vi "Calibrate In Ear.vi"(9 "Auto cal (F)?":bool, 11 "State":T1) -> (0 "error out":errorcluster)   [LabVIEW 2020]
uses:
  Utility VIs/Type Defs/Speaker ring.ctl
  Utility VIs/Buttons/KCheckmarkBoolean 2.ctl
  Cochlear Function Test Suite/LV Source/CFTS Main Panel SubVIs/CFTS-Experiment State.ctl
  Type Defs/ACal-In Ear Parameters.ctl
  Type Defs/Cal Stimulus.ctl
  Type Defs/ACal-Multiband Parameters.ctl
  Utility VIs/Conversion VIs/Create Waveform Cluster (2D).vi
  Utility VIs/Math VIs/FFT x(t) to dB,Degrees (2D).vi
  Instance           1 24Saved   Calibrate In Ear .vi
  Utility VIs/File IO VIs/Configuration File Wrapper VIs/Config-Read Key (Boolean).vi
panel:
  in  "Weighted":bool
  out "Auto Message":string="Auto calibrating!"
  in  "Speaker":T2
  in  "mic gain":dbl caption="Probe Mic Gain (dB)"
  in  "Stimulus":T3={"Min Freq (Hz)"=1000.0, "Max Freq (Hz)"=50000.0, "Freq Step (Hz)"=50.0, "Waveform"=0, "Attenuation (dB)"=30.0, "Sample Rate (Hz)"=100000.0} {"Waveform" items=["Chirp"]}
  out "Stimulus graph":cluster{i32, dbl, dbl[]}(graph)={0, 0.01, []}
  in  "Averages":i32=128
  in  "Return":bool
  in  "START":bool
  in  "STOP":bool
  out "Path":path
  in  "Data tab":enum32{"Raw", "Calibration"}(tab)
  out "Mic signals":cluster{"offset":dbl, "dx":dbl, "Y":dbl[][]}(graph)
  out "Mic mag":cluster{"offset":dbl, "dx":dbl, "Y":dbl[][]}(graph)
  out "Acquired":i32=256
  in  "Clear":bool
  in  "Load":bool
  in  "Show all":bool
  in  "Last N":bool
  out "ASTF":cluster{"Frequency":dbl[], "Frequency":dbl[]}[](graph)
  in  "Plot Max SPL":T4=TRUE
  in  "result":cluster{"Path":path, "error ":errorcluster}
  out "ASTF phase":cluster{"Frequency":dbl[], "Frequency":dbl[]}[](graph)
  out "Mic phase graph":cluster{"offset":dbl, "dx":dbl, "Y":dbl[][]}(graph)
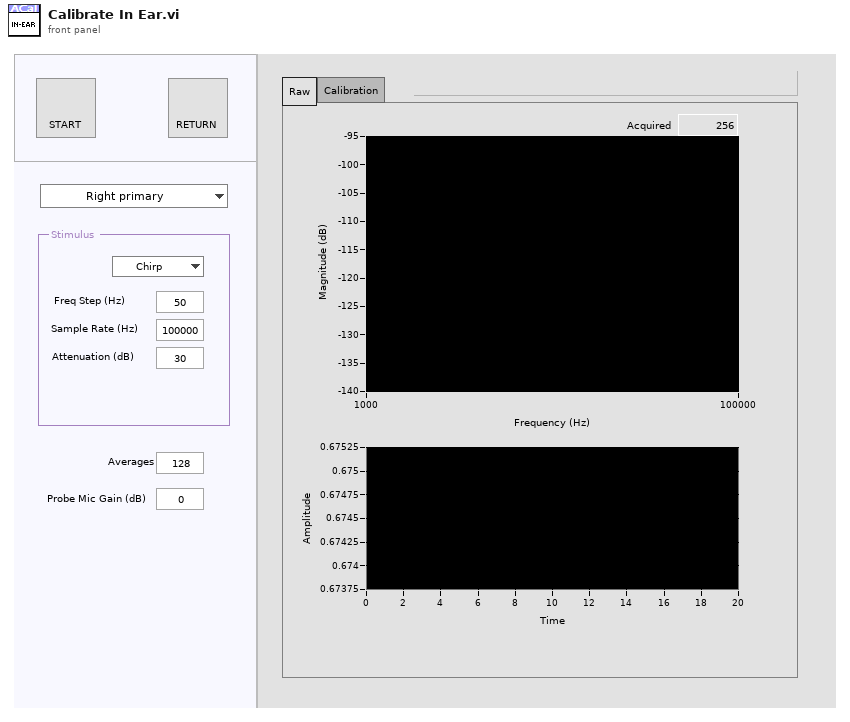
[diagram p1: front panel]
types:
  T1 = typedef "CFTS-Experiment State.ctl" = cluster{"Experimenter":string, "Number":u32, "Right":string, "Left":string, "Data Folder":path, "State File":path, "Version Info":string, "End Exposure Time":dbl, "Exposure Duration":string, "Run #":cluster{"CAP":i16, "ABR":i16, "DP":i16, "VsEP":i16, "MeasSeq":i16, "SubSeq":i16, "SFOAE":i16}}
  T2 = typedef "Speaker ring.ctl" = enum16{"Right primary", "Right secondary", "Left primary", "Left secondary"}
  T3 = cluster{"Min Freq (Hz)":dbl, "Max Freq (Hz)":dbl, "Freq Step (Hz)":dbl, "Waveform":u16, "Attenuation (dB)":dbl, "Sample Rate (Hz)":dbl}
  T4 = typedef "KCheckmarkBoolean 2.ctl" = bool
  T5 = typedef "ACal-In Ear Parameters.ctl" = cluster{"Speaker":T2, "Stimulus":T6, "Averages":i32, "Left gain":dbl, "Right gain":dbl, "plot max":bool, "smooth override":bool, "Weighted":T7, "Max Vmic":dbl}
  T6 = typedef "Cal Stimulus.ctl" = cluster{"Min Freq (Hz)":dbl, "Max Freq (Hz)":dbl, "Freq Step (Hz)":dbl, "Waveform":enum16{"Chirp", "Weighted"}, "Attenuation (dB)":dbl, "Sample Rate (Hz)":dbl}
  T7 = typedef "ACal-Multiband Parameters.ctl" = cluster{"Folder":path, "Fmin":dbl, "Fmax":dbl, "Max range":dbl, "WF":u16}
  T8 = typedef "Cal-Smoothing Parameters.ctl" = cluster{"Method":enum16{"None", "Moving average", "Loess"}, "MA":cluster{"Iterations":i32, "Length":i32}, "Loess":cluster{"Length":i32, "Type":enum16{"Linear", "Quadratic"}, "Robust":bool}}
  T9 = cluster{"new file path":path, "error out":errorcluster}
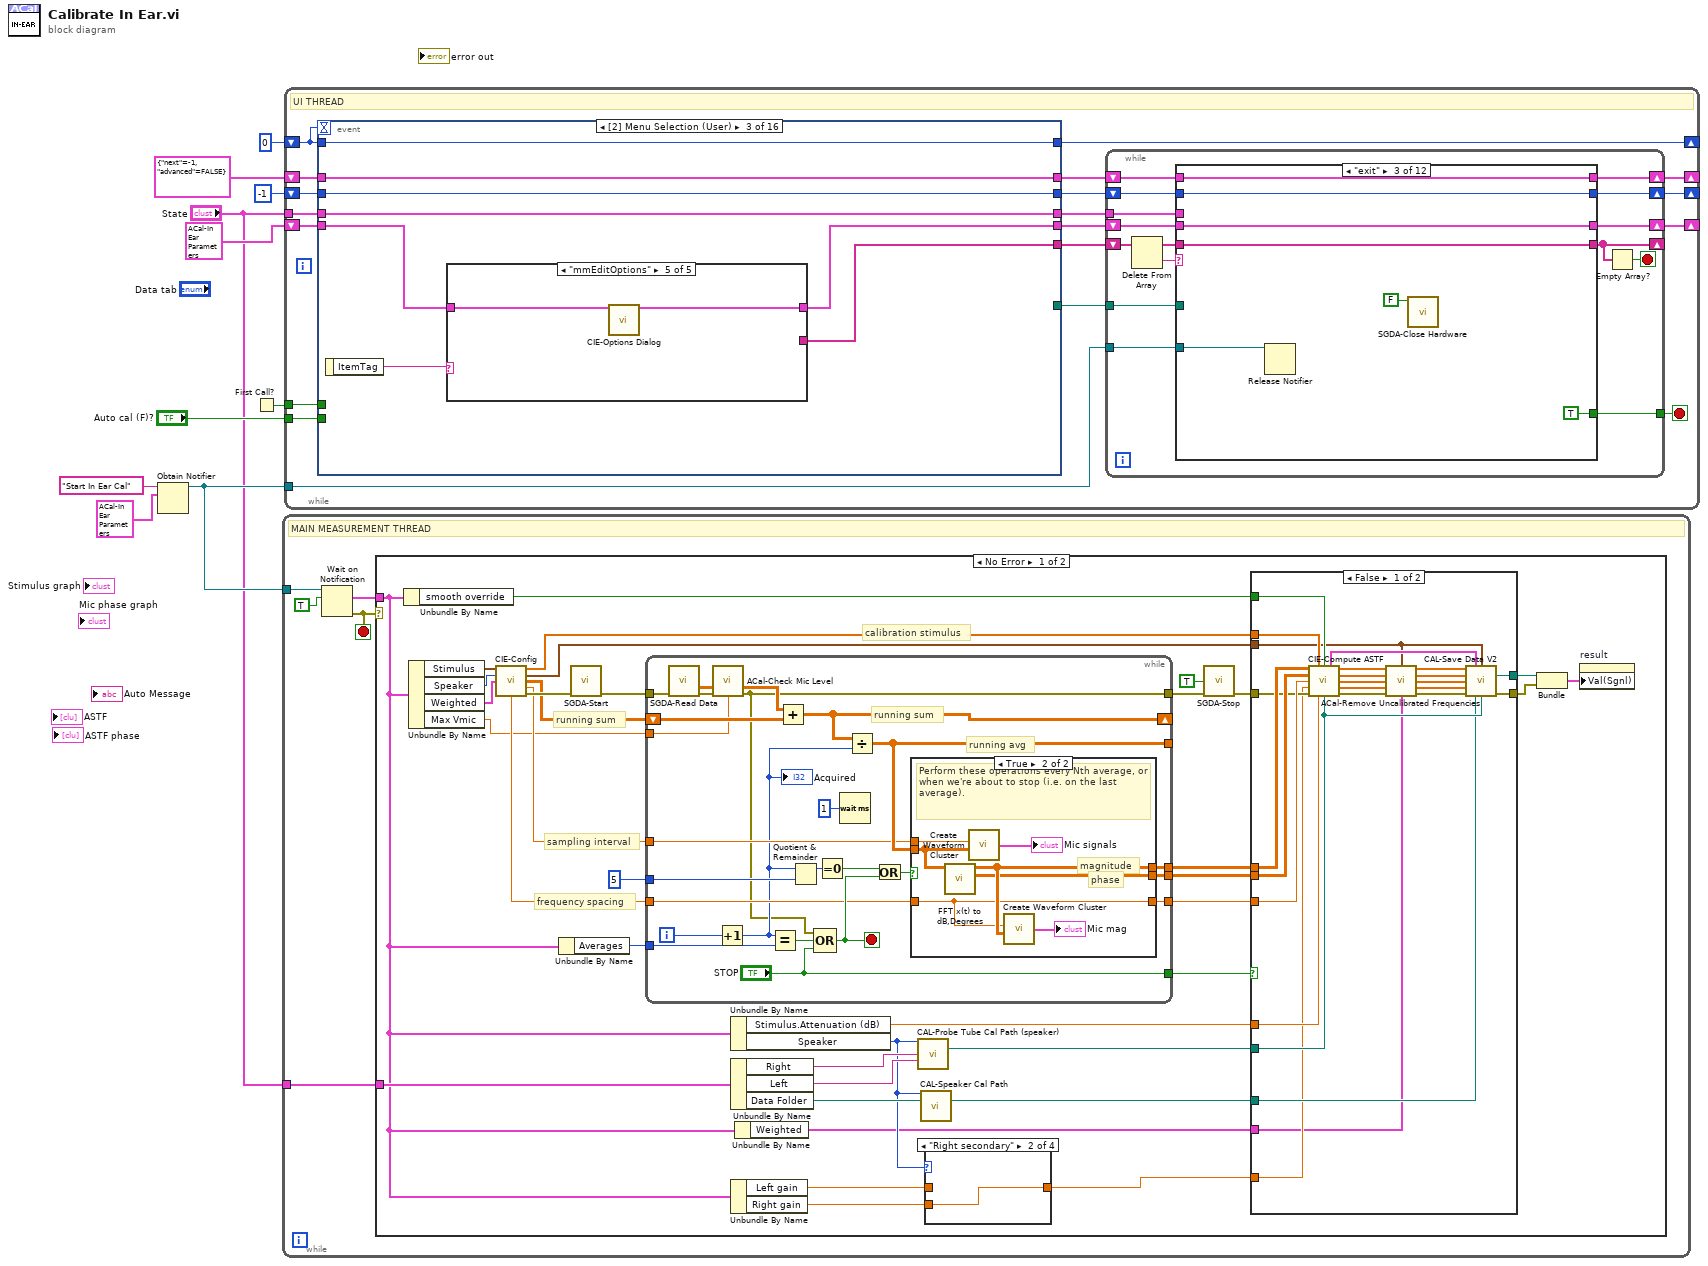
[diagram p0: block diagram]
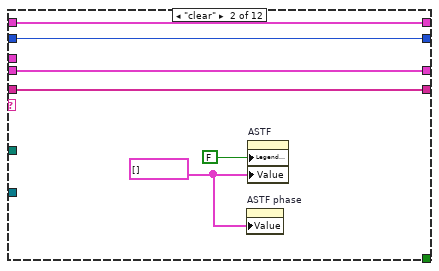
[diagram p9: hidden frame]
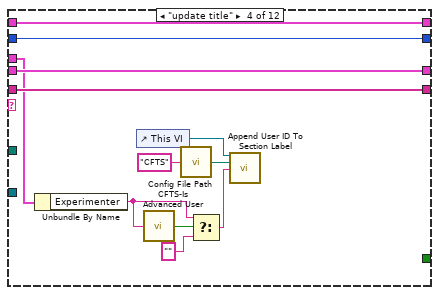
[diagram p10: hidden frame]
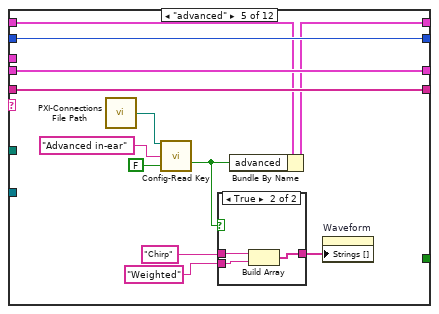
[diagram p11: hidden frame]
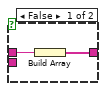
[diagram p12: hidden frame]
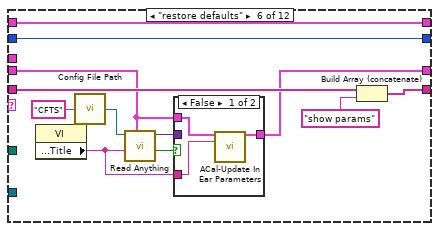
[diagram p13: hidden frame]
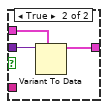
[diagram p14: hidden frame]
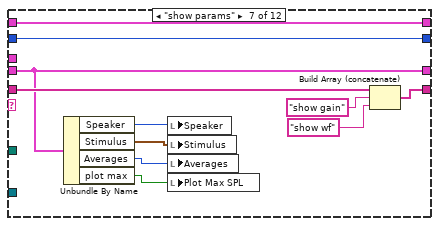
[diagram p15: hidden frame]
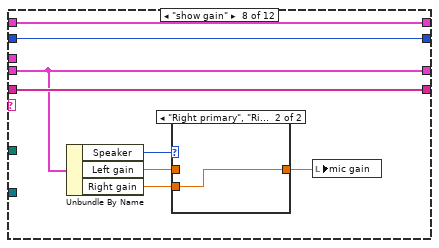
[diagram p16: hidden frame]
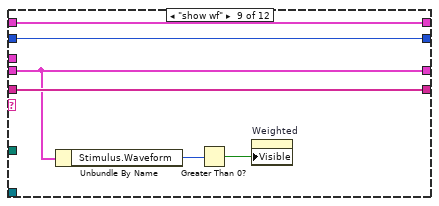
[diagram p18: hidden frame]
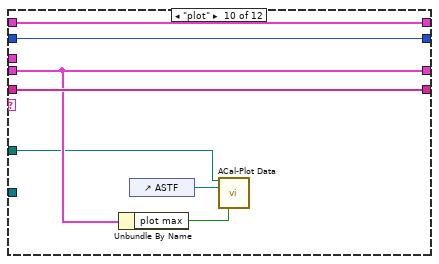
[diagram p19: hidden frame]
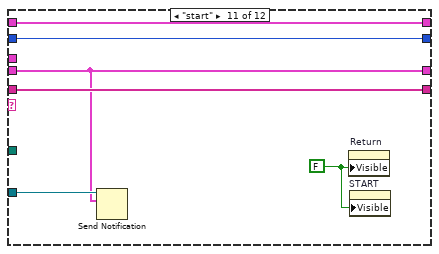
[diagram p20: hidden frame]
diagram:
  n1 = Obtain Notifier(name (unnamed)="Start In Ear Cal", notification data type=T5 {"Speaker"=enum."Right primary", "Stimulus"={"Min Freq (Hz)"=50.0, "Max Freq (Hz)"=50000.0, "Freq Step (Hz)"=50.0, "Waveform"=enum."Chirp", "Attenuation (dB)"=20.0, "Sample Rate (Hz)"=100000.0}, "Averages"=512, "Left gain"=40.0, "Right gain"=40.0, "plot max"=TRUE, "smooth override"=FALSE, "Weighted"={"Folder"=path "", "Fmin"=0.0, "Fmax"=0.0, "Max range"=0.0, "WF"=0}, "Max Vmic"=0.0} ("Params")) -> (notifier out=w10:refnum<notifier>)  [unwired: 2 in, 2 out]
  n2 = First Call?() -> (First Call?: T/F=w1:bool)
  n3 = while {
    tunnel: w10 -> [w15]
    tunnel: "State" -> [w13]
    stop <- w14 stop-if-true
    # "MAIN MEASUREMENT THREAD"
    n4 = Wait on Notification(notifier=w15, ignore previous (F)=TRUE) -> (notification=w12:T5, error out=w14:errorcluster)  [unwired: 2 in, 2 out]
    n5 = case shown="No Error" w14 {
      tunnel: w13 -> [w34 _]
      tunnel: w12 -> [w19 _]
      frame No Error {
        # "calibration stimulus"
        # "frequency spacing"
        # "sampling interval"
        # "running sum"
        n6 = Unbundle By Name(w19) -> ("smooth override"=w30:bool)
        n7 = Unbundle By Name(w19) -> ("Stimulus"=w33:T6, "Speaker"=w32:T2, "Weighted"=w20:T7, "Max Vmic"=w17:dbl)
        n8 = call "CIE-Config.vi"("Cal Stimulus"=w33, "Speaker"=w32, "Weighted"=w20) -> ("Stimulus"=w45:dbl[], "Cal Spec Out"=w36:T6, "Mic Avg"=w51:dbl[][], "dt (ms)"=w49:dbl, "df (Hz)"=w50:dbl, "error out"=w52:errorcluster)  [unwired: 6 in, 1 out]
        n9 = Unbundle By Name(w19) -> ("Averages"=w31:i32)
        n10 = call "SGDA-Start.vi"("error in (no error)"=w52) -> ("error out"=w44:errorcluster)  [unwired: 6 in]
        n11 = while {
          tunnel: w44 -> [w107]
          tunnel: [w83] -> w43
          tunnel: w31 -> [w104]
          shift-right: [w102] -> _
          shift-left: w51 -> [w103]
          tunnel: [w101] -> _
          tunnel: 5 -> [w100]
          tunnel: w50 -> [w95]
          tunnel: [w94] -> w48
          tunnel: [w93] -> w47
          tunnel: w49 -> [w92]
          tunnel: [w91] -> w46
          tunnel: ["STOP"] -> w28
          tunnel: w17 -> [w84]
          i -> [w106]
          stop <- w96 stop-if-true
          # "running avg"
          # "running sum"
          n12 = call "SGDA-Read Data.vi"("error in (no error)"=w107) -> ("AI Waveforms"=w86:dbl[][], "error out"=w87:errorcluster)  [unwired: 13 in]
          n13 = call "ACal-Check Mic Level.vi"("AI Waveforms in"=w86, "error in (no error)"=w87, "Max Vmic"=w84) -> ("AI Waveforms out"=w85:dbl[][], "error out"=w83:errorcluster)  [unwired: 11 in]
          n14 = Increment(x=w106) -> (x+1=w90:i32)
          "Acquired" <- w90
          n15 = Equal?(x=w90, y=w104) -> (x = y?=w105:bool)
          n16 = Add(x=w85, y=w103) -> (x+y=w102:dbl[][])
          n17 = Quotient & Remainder(x=w90, y=w100) -> (x-y*floor(x/y)=w99:i32)  [unwired: 1 out]
          n18 = Compound Arithmetic op=OR(w83, w105, "STOP") -> (w96:bool)
          n19 = Equal To 0?(x=w99) -> (x = 0?=w97:bool)
          n20 = Wait (ms)(milliseconds to wait=u32 1) -> ()  [unwired: 1 out]
          n21 = Divide(x=w102, y=w90) -> (x/y=w101:dbl[][])
          n22 = Or(x=w97, y=w96) -> (x .or. y?=w98:bool)
          n23 = case shown="True" w98 {
            tunnel: w101 -> [_ w111]
            tunnel: w95 -> [_ w108]
            tunnel: [_ w113] -> w94
            tunnel: [_ w112] -> w93
            tunnel: w92 -> [_ w110]
            tunnel: [_ w108] -> w91
            frame False {
            }
            frame True {
              # "phase"
              # "magnitude"
              # "Perform these operations every Nth average, or when we're about to stop (i.e. on the last average)."
              n24 = call-poly "FFT x(t) to dB,Degrees.vi"("X(t)"=w111) -> ("+Freq Phase of FFT (degrees)"=w112:dbl[][], "+Freq. Mag of FFT (dB rms)"=w113:dbl[][])  [unwired: 9 in]
              n25 = call-poly "Create Waveform Cluster.vi"("dx"=w110, "Array"=w111) -> ("waveform cluster"=→"Mic signals":cluster{"offset":dbl, "dx":dbl, "Y":dbl[][]})  [unwired: 3 in]
              n26 = call-poly "Create Waveform Cluster.vi"("dx"=w108, "Array"=w113) -> ("waveform cluster"=→"Mic mag":cluster{"offset":dbl, "dx":dbl, "Y":dbl[][]})  [unwired: 3 in]
            }
          }
        }
        n27 = Unbundle By Name(w19) -> ("Stimulus.Attenuation (dB)"=w29:dbl, "Speaker"=w27:T2)
        n28 = Unbundle By Name(w34) -> ("Right"=w41:string, "Left"=w40:string, "Data Folder"=w39:path)
        n29 = Unbundle By Name(w19) -> ("Left gain"=w26:dbl, "Right gain"=w24:dbl)
        n30 = Unbundle By Name(w19) -> ("Weighted"=w18:T7)
        n31 = call "CAL-Probe Tube Cal Path (speaker).vi"("Speaker"=w27, "Right"=w41, "Left"=w40) -> ("Probe Tube Cal Path"=w38:path)  [unwired: 11 in, 1 out]
        n32 = call "CAL-Speaker Cal Path.vi"("Speaker"=w27, "Data Folder"=w39) -> ("Cal Path"=w35:path)  [unwired: 12 in, 1 out]
        n33 = case shown="\"Right secondary\"" w27 {
          tunnel: w26 -> [_ _ w55 w56]
          tunnel: [w53 w54 w55 w56] -> w25
          tunnel: w24 -> [w53 w54 _ _]
          frame "Right primary", Default {
          }
          frame "Right secondary" {
          }
          frame "Left secondary" {
          }
          frame "Left primary" {
          }
        }
        n34 = call "SGDA-Stop.vi"("Clear ActiveX (F)"=TRUE, "error in (no error)"=w43) -> ("error out"=w37:errorcluster)  [unwired: 13 in]
        n35 = case shown="False" w28 {
          tunnel: w48 -> [w81 _]
          tunnel: w47 -> [w80 _]
          tunnel: w46 -> [w79 _]
          tunnel: w45 -> [w78 _]
          tunnel: w38 -> [w77 _]
          tunnel: w37 -> [w76 w82]
          tunnel: w36 -> [w58 _]
          tunnel: w35 -> [w74 _]
          tunnel: w30 -> [w73 _]
          tunnel: w29 -> [w72 _]
          tunnel: [w71 w82] -> w22
          tunnel: [w70 _] -> w23
          tunnel: w25 -> [w69 _]
          tunnel: w18 -> [w57 _]
          frame False {
            n36 = call "CIE-Compute ASTF.vi"("Mag"=w81, "Stimulus"=w78, "Force no smoothing?"=w73, "Phase"=w80, "df (Hz)"=w79, "Probe Mic Gain (dB)"=w69, "error in (no error)"=w76, "Attenuation (dB)"=w72, "Probe Tube Path"=w77) -> ("Smooth Params"=w75:T8, "ASTF Mag"=w60:dbl[], "ASTF Phase"=w61:dbl[], "Frequency"=w64:dbl[], "Unsmoothed Mag"=w65:dbl[], "error out"=w68:errorcluster)  [unwired: 1 in]
            n37 = call "ACal-Remove Uncalibrated Frequencies.vi"("ASTF Mag in"=w60, "Cal Spec Out"=w58, "ASTF Phase in"=w61, "Frequency in"=w64, "Unsmoothed Mag in"=w65, "error in (no error)"=w68, "Weighted"=w57) -> ("ASTF Mag out"=w59:dbl[], "ASTF Phase out"=w62:dbl[], "Frequency out"=w63:dbl[], "Unsmoothed Mag out"=w66:dbl[], "error out"=w67:errorcluster)  [unwired: 4 in]
            n38 = call "CAL-Save Data V2.vi"("Mag"=w59, "Smooth Params"=w75, "Cal Stimulus"=w58, "Phase"=w62, "Frequency"=w63, "Unsmoothed Mag"=w66, "error in (no error)"=w67, "path"=w74, "Probe Tube File"=w77) -> ("new file path"=w70:path, "error out"=w71:errorcluster)  [unwired: 5 in]
          }
          frame True {
          }
        }
        n39 = Bundle("new file path"=w23, "error out"=w22) -> (w21:T9)  [unwired: 1 in]
        n40 = property on="result" class="Clust (strict)"("Val(Sgnl)"=w21) -> ()  [unwired: 2 in, 2 out]
      }
      frame Error {
      }
    }
  }
  n41 = while {
    tunnel: w10 -> [w121]
    shift-right: [w130] -> _
    shift-left: 0 -> [w131]
    tunnel: "Auto cal (F)?" -> [w133]
    shift-right: [w124] -> _
    shift-left: -1 -> [w132]
    tunnel: "State" -> [w129]
    shift-right: [w125] -> _
    shift-left: T5 {"Speaker"=enum."Right primary", "Stimulus"={"Min Freq (Hz)"=50.0, "Max Freq (Hz)"=50000.0, "Freq Step (Hz)"=50.0, "Waveform"=enum."Chirp", "Attenuation (dB)"=20.0, "Sample Rate (Hz)"=100000.0}, "Averages"=512, "Left gain"=40.0, "Right gain"=40.0, "plot max"=TRUE, "smooth override"=FALSE, "Weighted"={"Folder"=path "C:/Data", "Fmin"=3000.0, "Fmax"=45000.0, "Max range"=25.0, "WF"=0}, "Max Vmic"=0.0} ("Params") -> [w128]
    shift-right: [w116] -> _
    shift-left: cluster{"next":i32, "advanced":bool} {"next"=-1, "advanced"=FALSE} -> [w118]
    tunnel: w1 -> [w115]
    stop <- w122 stop-if-true
    # "UI THREAD"
    n42 = event shown="[2] Menu Selection (User)" {
      selector: _ -> [_ _ _ _ _ _ _ _ _ _ _ _ _ _ _ _]
      dyn-events: _ -> [_ _ _ _ _ _ _ _ _ _ _ _ _ _ _ _]
      timeout: w131 -> [_ _ _ _ _ _ _ _ _ _ _ _ _ _ _ _]
      tunnel: w133 -> [w288 _ _ _ _ _ _ _ _ _ _ w411 _ _ _ _]
      tunnel: w132 -> [w289 w306 w315 w335 w342 w350 w353 w366 w368 w381 w394 w419 w435 w442 w457 w467]
      tunnel: [w289 w306 w315 w335 w342 w350 w353 w366 w368 w381 w394 w419 w435 w442 w457 w467] -> w127
      tunnel: w131 -> [_ w305 w314 w334 w341 w349 w358 w365 w373 w380 w393 w418 w434 w441 w455 w465]
      tunnel: [-1 w305 w314 w334 w341 w349 w358 w365 w373 w380 w393 w418 w434 w441 w455 w465] -> w130
      tunnel: w129 -> [w284 w302 w309 w331 w340 w344 w356 w364 w371 w376 w391 w416 w431 w439 w454 w464]
      tunnel: w128 -> [w286 w304 w312 w333 w339 w348 w357 w362 w372 w378 w392 w417 w433 w440 w453 w463]
      tunnel: [w286 w304 w311 w333 w339 w346 w355 w360 w370 w377 w390 w417 w433 w440 w453 w463] -> w126
      tunnel: [w283 string[] ["exit"] w310 string[] ["exit"] string[] ["start"] string[] ["show gain"] string[] ["show wf"] _ _ _ _ w409 string[] ["clear"] w437 _ _] -> w123
      tunnel: [w284 w302 w309 w331 w340 w344 w356 w364 w371 w376 w391 w416 w431 w439 w454 w464] -> w120
      tunnel: [_ _ _ _ _ _ _ _ _ _ _ w414 _ w438 _ _] -> w119
      tunnel: w118 -> [w281 w301 w308 w330 w338 w343 w352 w363 w367 w374 w388 w413 w430 w436 w451 w460]
      tunnel: [w281 w301 w308 w330 w338 w343 w352 w363 w367 w374 w388 w413 w430 w436 w451 w460] -> w117
      tunnel: w115 -> [w279 _ _ _ _ _ _ _ _ _ _ _ _ _ _ _]
      event Timeout {
        w295 = TRUE ("Visible")
        n43 = event-data() -> ()  [unwired: 1 in, 1 out]
        n44 = call "SGDA-Initialize Hardware.vi"("Start PXI Server"=FALSE) -> ()  [unwired: 13 in, 2 out]
        n45 = case shown="False" w288 {
          tunnel: [w297 string[] ["next", "clear"]] -> w285
          tunnel: w279 -> [w299 _]
          frame False {
            n46 = Select(t=string[] ["clear"], s=w299, f=string[] []) -> (s? t:f=w297:string[])
          }
          frame True {
          }
        }
        n47 = property on="Auto Message" class="Str"("Visible"=w288, "Blinking"=w288) -> ()  [unwired: 2 in, 2 out]
        n48 = Unbundle By Name(w284) -> ("Experimenter"=w294:string)
        n49 = property on="Weighted" class="Bool"("Visible"=FALSE) -> ()  [unwired: 2 in, 2 out]
        n50 = Concatenate Strings(w294, ": Last 5" ("string")) -> (w292:string)
        n51 = property on="START" class="Bool"("Visible"=w295) -> ()  [unwired: 2 in, 2 out]
        n52 = property on="Return" class="Bool"("Visible"=w295) -> ()  [unwired: 2 in, 2 out]
        n53 = Initialize Array(w292, 4 ("dimension size")) -> (w290:string[])
        n54 = property on="Last N" class="Bool"("Strings [4]"=w290) -> ()  [unwired: 2 in, 2 out]
        n55 = Build Array (concatenate)(w285, string[] ["restore defaults", "advanced", "update title"]) -> (w283:string[])
      }
      event Panel Close? {
        n56 = event-data() -> ()  [unwired: 1 in, 1 out]
        n57 = event-data("Discard?"=TRUE) -> ()  [unwired: 1 in, 1 out]
      }
      event Menu Selection (User) {
        n58 = event-data() -> ("ItemTag"=w313:string)  [unwired: 1 in]
        n59 = case shown="\"mmEditOptions\"" w313 {
          tunnel: w312 -> [w316 w318 w321 w327 w329]
          tunnel: [w316 w318 w321 w327 w328] -> w311
          tunnel: [_ string[] ["restore defaults"] _ string[] ["exit"] _] -> w310
          frame "", Default {
          }
          frame "mmFileRestore" {
          }
          frame "mmFileSave" {
            n60 = property class="VI"() -> ("Front Panel.Title"=w320:string)  [unwired: 2 in, 2 out]
            n61 = call "Config File Path.vi"("AppName"="CFTS") -> ("Default config file name"=w322:path)
            n62 = call "Write Anything.vi"("Section Name (Name of \"Anything\")"=w320, "Anything"=w321, "Path (dialog)"=w322) -> ("Error Out"=w319:errorcluster)  [unwired: 7 in, 1 out]
            n63 = case shown="Error" w319 {
              selector: w319 -> [_ w325]
              frame No Error {
                n64 = One Button Dialog(message="Defaults saved.") -> ()  [unwired: 1 in, 1 out]
              }
              frame Error {
                n65 = call "Error Handler.vi"("error in (no error)"=w325) -> ()  [unwired: 13 in, 2 out]
              }
            }
          }
          frame "mmFileExit" {
          }
          frame "mmEditOptions" {
            n66 = call "CIE-Options Dialog.vi"("Override smoothing"=w329) -> ("Override Out"=w328:T5)  [unwired: 13 in, 1 out]
          }
        }
      }
      event "Return": Value Change {
        n67 = event-data() -> ()  [unwired: 1 in, 1 out]
      }
      event "START": Value Change {
        n68 = event-data() -> ()  [unwired: 1 in, 1 out]
        n69 = local write "Data tab"(enum32{"Raw", "Calibration"}."Raw" ("Data tab")) -> ()
      }
      event Value Change {
        n70 = event-data() -> ("NewVal"=w345:T2)  [unwired: 1 in]
        n71 = Bundle By Name(cluster=w348, "Speaker"=w345) -> (w346:T5)
      }
      event "Stimulus": Value Change {
        n72 = event-data() -> ()  [unwired: 1 in, 1 out]
        n73 = Bundle By Name(cluster=w357, "Stimulus"="Stimulus") -> (w355:T5)
      }
      event "Weighted": Value Change {
        n74 = event-data() -> ()  [unwired: 1 in, 1 out]
        n75 = Unbundle By Name(w362) -> ("Weighted"=w361:T7)
        n76 = call "ACal-Multiband Dialog.vi"("Cluster In"=w361) -> ("Cluster out"=w359:T7)  [unwired: 13 in, 1 out]
        n77 = Bundle By Name(cluster=w362, "Weighted"=w359) -> (w360:T5)
      }
      event "Averages": Value Change {
        n78 = event-data() -> ()  [unwired: 1 in, 1 out]
        n79 = Bundle By Name(cluster=w372, "Averages"="Averages") -> (w370:T5)
      }
      event "mic gain": Value Change {
        n80 = event-data() -> ()  [unwired: 1 in, 1 out]
        n81 = Unbundle By Name(w378) -> ("Speaker"=w379:T2)
        n82 = case shown="\"Right primary\", \"Right secondary\"" w379 {
          tunnel: w378 -> [w384 w387]
          tunnel: [w383 w386] -> w377
          tunnel: "mic gain" -> [w382 w385]
          frame "Left primary", Default {
            n83 = Bundle By Name(cluster=w384, "Left gain"=w382) -> (w383:T5)
          }
          frame "Right primary", "Right secondary" {
            n84 = Bundle By Name(cluster=w387, "Right gain"=w385) -> (w386:T5)
          }
        }
      }
      event Value Change {
        # "Clear the plot because the scaling is no longer consistent with the option. We haven't retained a list of displayed data files, so we can't restore them with the proper scaling. The best we can do (without more serious revision) is to reload the last saved calibration file."
        n85 = event-data() -> ("NewVal"=w399:T4)  [unwired: 1 in]
        n86 = control-ref of="ASTF"() -> (w397:refnum<vi>)
        n87 = property class="XYGraph (strict)"(reference=w397, "Value"=cluster{"Frequency":dbl[], "Frequency":dbl[]}[] []) -> (reference out=w395:refnum<vi>, error out=w398:errorcluster)  [unwired: 1 in]
        n88 = Bundle By Name(cluster=w392, "plot max"="Plot Max SPL") -> (w390:T5)
        n89 = local read "Path"() -> (w401:path)
        n90 = call "FileIO-File or Folder Exists.vi"("error in (no error)"=w398, "path"=w401) -> ("Directory?"=w402:bool, "dup path"=w400:path)  [unwired: 6 in, 2 out]
        n91 = case shown="True" w402 {
          tunnel: w395 -> [_ w405]
          tunnel: w399 -> [_ w403]
          tunnel: w400 -> [_ w406]
          frame False {
          }
          frame True {
            n92 = call "ACal-Plot Data.vi"("Path"=w406, "Mag graph"=w405, "Plot max"=w403) -> ("error out"=w404:errorcluster)  [unwired: 11 in, 1 out]
            n93 = call <vilib>:"Simple Error Handler.vi"("error in (no error)"=w404) -> ()  [unwired: 4 in, 5 out]
          }
        }
      }
      event "result": Value Change {
        w412 = TRUE
        n94 = event-data() -> ("NewVal.Path"=w415:path, "NewVal.error"=w408:errorcluster)  [unwired: 1 in]
        n95 = call "Beeper.vi"() -> ()  [unwired: 5 in, 1 out]
        n96 = case shown="No Error" w408 {
          selector: w408 -> [_ w429]
          tunnel: w415 -> [w428 _]
          tunnel: [w428 _] -> w414
          tunnel: [w425 _] -> w410
          frame No Error {
            n97 = Empty String/Path?(string/path=w428) -> (empty?=w427:bool)
            n98 = Select(t=string[] [], s=w427, f=string[] ["plot"]) -> (s? t:f=w425:string[])
            "Path" <- w428
          }
          frame Error {
            n99 = call "Error Handler.vi"("error in (no error)"=w429) -> ()  [unwired: 13 in, 2 out]
          }
        }
        n100 = case shown="False" w411 {
          tunnel: w410 -> [w420 w423]
          tunnel: [w420 w422] -> w409
          frame False {
          }
          frame True {
            n101 = Build Array (concatenate)("next", w423) -> (w422:string[])
          }
        }
        n102 = local write "Data tab"(enum32{"Raw", "Calibration"}."Calibration" ("Data tab")) -> ()
        n103 = property on="START" class="Bool"("Visible"=w412) -> ()  [unwired: 2 in, 2 out]
        n104 = property on="Return" class="Bool"("Visible"=w412) -> ()  [unwired: 2 in, 2 out]
      }
      event "Clear": Value Change {
        n105 = event-data() -> ()  [unwired: 1 in, 1 out]
      }
      event "Load": Value Change {
        n106 = event-data() -> ()  [unwired: 1 in, 1 out]
        n107 = Unbundle By Name(w439) -> ("Data Folder"=w443:path)
        n108 = call "File Dialog"("start path"=w443, "pattern (all files)"="*.calib", "pattern label"="Calibration files") -> ("selected path"=w448:path, "cancelled"=w447:bool, "error out"=w446:errorcluster)  [unwired: 9 in, 1 out]
        n109 = case shown="False" w447 {
          tunnel: w448 -> [w450 _]
          tunnel: w446 -> [_ _]
          tunnel: [w450 _] -> w438
          tunnel: [string[] ["plot"] _] -> w437
          frame False {
          }
          frame True {
          }
        }
      }
      event "Show all": Value Change {
        n110 = event-data() -> ()  [unwired: 1 in, 1 out]
        n111 = Unbundle By Name(w453) -> ("plot max"=w452:bool)
        n112 = Unbundle By Name(w454) -> ("Data Folder"=w458:path)
        n113 = control-ref of="ASTF"() -> (w456:refnum<vi>)
        n114 = call "CAL-Show all.vi"("Path"=w458, "Mag graph"=w456, "Plot Max SPL"=w452) -> ("error out"=w459:errorcluster)  [unwired: 11 in, 1 out]
        n115 = call "Error Handler.vi"("error in (no error)"=w459) -> ()  [unwired: 13 in, 2 out]
      }
      event "Last N": Value Change {
        n116 = event-data() -> ()  [unwired: 1 in, 1 out]
        n117 = Unbundle By Name(w463) -> ("Speaker"=w461:T2, "plot max"=w462:bool)
        n118 = control-ref of="ASTF"() -> (w466:refnum<vi>)
        n119 = call "CAL-Show Last N.vi"("Expt State"=w464, "Mag graph"=w466, "Speaker"=w461, "Plot Max SPL"=w462) -> ("error out"=w468:errorcluster)  [unwired: 11 in]
        n120 = call <vilib>:"Simple Error Handler.vi"("error in (no error)"=w468) -> ()  [unwired: 4 in, 5 out]
      }
    }
    n121 = while {
      shift-right: [w146] -> w125
      shift-left: w126 -> [w147]
      shift-right: [w145] -> w124
      shift-left: w127 -> [w148]
      shift-right: [w141] -> _
      shift-left: w123 -> [w143]
      tunnel: w121 -> [w139]
      tunnel: [w138] -> w122
      tunnel: w120 -> [w137]
      tunnel: w119 -> [w136]
      shift-right: [w135] -> w116
      shift-left: w117 -> [w134]
      stop <- w140 stop-if-true
      n122 = Delete From Array(array=w143) -> (deleted portion=w142:string, array with subset deleted=w144:string[])  [unwired: 2 in]
      n123 = case shown="\"exit\"" w142 {
        tunnel: w148 -> [w152 w158 w165 w177 w189 w206 w223 w231 w239 w246 w252 w265]
        tunnel: [w152 w158 w165 w177 w189 w206 w223 w231 w239 w246 w252 w265] -> w145
        tunnel: w147 -> [w151 w157 w164 w176 w188 w201 w221 w229 w236 w244 w247 w258]
        tunnel: [w151 w157 w164 w176 w188 w200 w221 w229 w236 w244 w247 w257] -> w146
        tunnel: w144 -> [w150 w156 w163 w175 w187 w205 w222 w230 w238 w245 w248 w256]
        tunnel: [w150 w156 w163 w175 w187 w199 w216 w230 w238 w245 w248 w253] -> w141
        tunnel: w139 -> [_ _ w162 _ _ _ _ _ _ _ w249 _]
        tunnel: [_ _ TRUE _ _ _ _ _ _ _ _ w261] -> w138
        tunnel: w137 -> [_ _ _ w168 _ _ _ _ _ _ _ _]
        tunnel: w136 -> [_ _ _ _ _ _ _ _ _ w241 _ _]
        tunnel: [w149 w153 w160 w166 w182 w195 w214 w224 w237 w240 w251 w254] -> w135
        tunnel: w134 -> [w149 w153 w160 w166 w183 w195 w214 w224 w237 w240 w251 w255]
        frame "", Default {
        }
        frame "clear" {
          w155 = cluster{"Frequency":dbl[], "Frequency":dbl[]}[] [] ("ASTF mag")
          n124 = property on="ASTF phase" class="XYGraph (strict)"("Value"=w155) -> ()  [unwired: 2 in, 2 out]
          n125 = property on="ASTF" class="XYGraph (strict)"("Legend Visible"=FALSE ("Legend:Visible"), "Value"=w155) -> ()  [unwired: 2 in, 2 out]
        }
        frame "exit" {
          n126 = Release Notifier(notifier=w162) -> ()  [unwired: 2 in, 3 out]
          n127 = call "SGDA-Close Hardware.vi"("Stop PXI Server (T)"=FALSE) -> ()  [unwired: 6 in, 1 out]
        }
        frame "update title" {
          n128 = Unbundle By Name(w168) -> ("Experimenter"=w167:string)
          n129 = control-ref of="This VI"() -> (w169:refnum<vi>)
          n130 = call "CFTS-Is Advanced User.vi"("Experimenter"=w167) -> ("Advanced user"=w172:bool)
          n131 = call "Config File Path.vi"("AppName"="CFTS") -> ("Default config file name"=w170:path)
          n132 = Select(t=w167, s=w172, f="") -> (s? t:f=w174:string)
          n133 = call "Append User ID To Section Label.vi"("VI reference"=w169, "Path (dialog)"=w170, "User"=w174) -> ()  [unwired: 9 in, 4 out]
        }
        frame "advanced" {
          n134 = call "PXI-Connections File Path.vi"() -> ("Path"=w184:path)  [unwired: 1 in]
          n135 = call-poly "Config-Read Key.vi"("configuration file path"=w184, "key"="Advanced in-ear", "default"=FALSE) -> ("value"=w181:bool)  [unwired: 9 in, 3 out]
          n136 = case shown="True" w181 {
            tunnel: "Chirp" ("key") -> [w191 w194]
            tunnel: "Weighted" ("key") -> [_ w193]
            tunnel: [w190 w192] -> w178
            frame False {
              n137 = Build Array(w191) -> (w190:string[])
            }
            frame True {
              n138 = Build Array(w194, w193) -> (w192:string[])
            }
          }
          n139 = Bundle By Name(cluster=w183, "advanced"=w181) -> (w182:cluster{"next":i32, "advanced":bool})
          n140 = property on="Waveform" class="Ring (strict)"("Strings []"=w178) -> ()  [unwired: 2 in, 2 out]
        }
        frame "restore defaults" {
          n141 = property class="VI"() -> ("Front Panel.Title"=w197:string)  [unwired: 2 in, 2 out]
          n142 = call "Config File Path.vi"("AppName"="CFTS") -> ("Default config file name"=w196:path)
          n143 = call "Read Anything.vi"("Type of Anything"=w201, "Section Name (Name of \"Type of Anything\")"=w197, "Path (dialog)"=w196) -> ("Found?"=w203:bool, "Anything"=w202:variant)  [unwired: 6 in, 1 out]
          n144 = case shown="False" w203 {
            tunnel: w202 -> [_ w212]
            tunnel: w201 -> [w209 w211]
            tunnel: [w208 w210] -> w200
            tunnel: w197 -> [w207 _]
            frame False {
              n145 = call "ACal-Update In Ear Parameters.vi"("Params in"=w209, "Section"=w207) -> ("Params out"=w208:T5)  [unwired: 13 in]
            }
            frame True {
              n146 = Variant To Data(type=w211, Variant=w212) -> (data=w210:T5)  [unwired: 1 in, 1 out]
            }
          }
          n147 = Build Array (concatenate)(w205, "show params") -> (w199:string[])
        }
        frame "show params" {
          n148 = Unbundle By Name(w221) -> ("Speaker"=w220:T2, "Stimulus"=w219:T6, "Averages"=w218:i32, "plot max"=w217:bool)
          n149 = local write "Speaker"(w220) -> ()
          n150 = local write "Stimulus"(w219) -> ()
          n151 = local write "Averages"(w218) -> ()
          n152 = local write "Plot Max SPL"(w217) -> ()
          n153 = Build Array (concatenate)(w222, "show gain", "show wf") -> (w216:string[])
        }
        frame "show gain" {
          n154 = Unbundle By Name(w229) -> ("Speaker"=w227:T2, "Left gain"=w226:dbl, "Right gain"=w225:dbl)
          n155 = case shown="\"Right primary\", \"Right secondary\"" w227 {
            tunnel: w226 -> [w232 _]
            tunnel: w225 -> [_ w233]
            tunnel: [w232 w233] -> w228
            frame "Left primary", Default {
            }
            frame "Right primary", "Right secondary" {
            }
          }
          n156 = local write "mic gain"(w228) -> ()
        }
        frame "show wf" {
          n157 = Unbundle By Name(w236) -> ("Stimulus.Waveform"=w235:enum16{"Chirp", "Weighted"})
          n158 = Greater Than 0?(x=w235) -> (x > 0?=w234:bool)
          n159 = property on="Weighted" class="Bool"("Visible"=w234) -> ()  [unwired: 2 in, 2 out]
        }
        frame "plot" {
          n160 = Unbundle By Name(w244) -> ("plot max"=w243:bool)
          n161 = control-ref of="ASTF"() -> (w242:refnum<vi>)
          n162 = call "ACal-Plot Data.vi"("Path"=w241, "Mag graph"=w242, "Plot max"=w243) -> ()  [unwired: 11 in, 2 out]
        }
        frame "start" {
          w250 = FALSE
          n163 = Send Notification(notification=w247, notifier=w249) -> ()  [unwired: 1 in, 2 out]
          n164 = property on="Return" class="Bool"("Visible"=w250) -> ()  [unwired: 2 in, 2 out]
          n165 = property on="START" class="Bool"("Visible"=w250) -> ()  [unwired: 2 in, 2 out]
        }
        frame "next" {
          w260 = T2[] [enum."Right primary", enum."Right secondary", enum."Left primary", enum."Left secondary"] items=["Right primary", "Right secondary", "Left primary", "Left secondary"]
          n166 = Unbundle By Name(w255) -> ("next"=w264:i32)
          n167 = Array Size(array=w260) -> (size(s)=w263:i32)
          n168 = Increment(x=w264) -> (x+1=w259:i32)
          n169 = Less?(x=w259, y=w263) -> (x < y?=w262:bool)
          n170 = case shown="True" w262 {
            tunnel: [TRUE _] -> w261
            tunnel: w260 -> [_ w277]
            tunnel: w259 -> [_ w272]
            tunnel: w258 -> [w268 w276]
            tunnel: [w268 w274] -> w257
            tunnel: [w267 string[] ["start"]] -> w253
            tunnel: w256 -> [w267 _]
            tunnel: w255 -> [w266 w273]
            tunnel: [w266 w271] -> w254
            frame False {
            }
            frame True {
              n171 = Index Array(array=w277, index=w272) -> (element=w275:T2)
              n172 = Bundle By Name(cluster=w276, "Speaker"=w275) -> (w274:T5)
              n173 = local write "Speaker"(w275) -> ()
              n174 = Bundle By Name(cluster=w273, "next"=w272) -> (w271:cluster{"next":i32, "advanced":bool})
            }
          }
        }
      }
      n175 = Empty Array?(array=w141) -> (empty?=w140:bool)
    }
  }
